vi "run script line.vi"(8 "error in (no error)":errorcluster caption="에러 입력(에러 없음)", 11 "Script Line_gpio 입력":refnum<class "Script Line_gpio.lvclass">) -> (0 "error out":errorcluster caption="에러 출력", 2 "log":string, 3 "Script Line_gpio 출력":refnum<class "Script Line_gpio.lvclass">)   [LabVIEW 2020, in "Script Line_gpio.lvclass"]
uses:
  Script Line_gpio.lvclass
  SubVIs/GPIO/Controls/(Ctrl)GPIO_FGV Enum.ctl
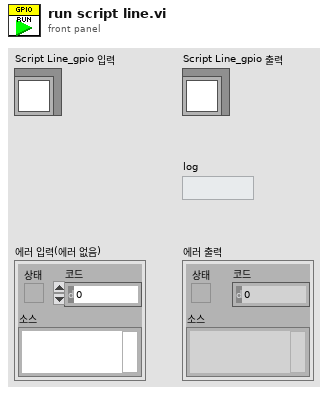
[diagram p1: front panel]
types:
  T1 = typedef "(Ctrl)GPIO_FGV Enum.ctl" = enum16{"Read Status", "GPIO Control", "Register Ctrl Ref"}
  T2 = typedef "(Ctrl)System Command_GPIO Control.ctl" = cluster{"Pin No.":u8, "Status":bool}
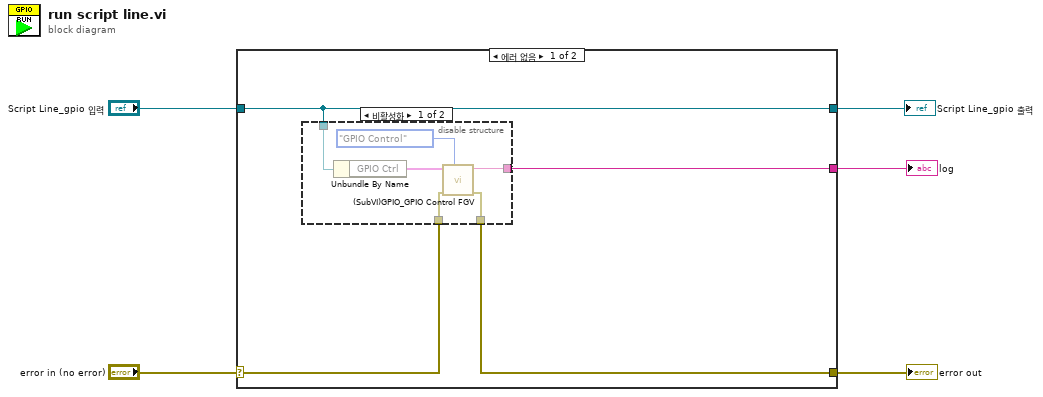
[diagram p0: block diagram]
diagram:
  n1 = case shown="에러 없음" "error in (no error)" {
    selector: "error in (no error)" -> [w7 w17]
    tunnel: [w6 w17] -> w5
    tunnel: [w9 w16] -> w4
    tunnel: "Script Line_gpio 입력" -> [w9 w16]
    tunnel: [w8 _] -> w1
    frame No Error {
      n2 = disable-structure shown="비활성화" {
        disable-tunnel: w9 -> [w15 _]
        disable-tunnel: [w12 _] -> w8
        disable-tunnel: w7 -> [w11 _]
        disable-tunnel: [w10 _] -> w6
        frame Disabled {
          n3 = Unbundle By Name(w15) -> ("GPIO Ctrl"=w14:T2[])
          n4 = call "(SubVI)GPIO_GPIO Control FGV.vi"("Function"=(Ctrl)GPIO_FGV_Enum."GPIO Control", "error in (no error)"=w11, "GPIO Ctrl"=w14) -> ("error out"=w10:errorcluster, "Log"=w12:string)  [unwired: 7 in]
        }
        frame Enabled {
        }
      }
    }
    frame Error {
    }
  }
  "error out" <- w5
  "Script Line_gpio 출력" <- w4
  "log" <- w1
